vi "Enable B output.vi"(8 "error in (no error)":errorcluster, 11 "Sync Box in":refnum<class "Sync Box.lvclass">) -> (0 "error out":errorcluster, 3 "Sync Box out":refnum<class "Sync Box.lvclass">)   [LabVIEW 2018, in "Sync Box.lvclass"]
uses:
  Sync Box.lvclass
  Sync Box.lvclass/Sync Box.ctl
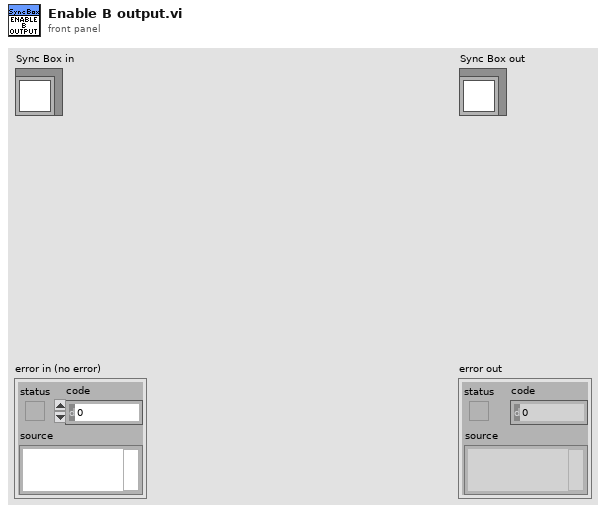
[diagram p1: front panel]
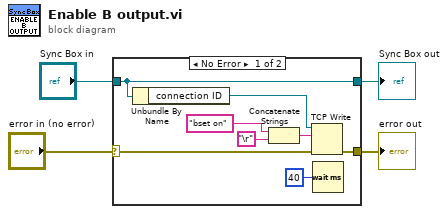
[diagram p0: block diagram]
diagram:
  n1 = case shown="No Error" "error in (no error)" {
    selector: "error in (no error)" -> [w10 w14]
    tunnel: [w9 w14] -> w1
    tunnel: "Sync Box in" -> [w6 w13]
    tunnel: [w6 w13] -> w2
    frame No Error {
      n2 = Unbundle By Name(w6) -> ("connection ID"=w7:refnum<k5>)
      n3 = Concatenate Strings("bset on", "\r") -> (w12:string)
      n4 = TCP Write(connection ID=w7, data in=w12, error in (no error)=w10) -> (error out=w9:errorcluster)  [unwired: 1 in, 2 out]
      n5 = Wait (ms)(milliseconds to wait=u32 40) -> ()  [unwired: 1 out]
    }
    frame Error {
    }
  }
  "error out" <- w1
  "Sync Box out" <- w2
